vi "PWM2 Init.vi"(5 "DutyCycle":u16, 6 "Precision":u16, 7 "Polarity":u8, 9 "Frequency":u32, 10 "ChannelIndex":u8, 11 "DevHandle":i32) -> (3 "function return":i32)   [LabVIEW 2010, in "usb2pwm.lvlib"]
doc: "int WINAPI PWM2_Init(int DevHandle, unsigned char ChannelIndex,unsigned int Frequency, unsigned char Polarity,unsigned short Precision, unsigned short DutyCycle);"
uses:
  usb2pwm.lvlib
  USB2XXX/trunk/USB2XXX/USB2XXX/vs2019/Release/USB2XXX.dll
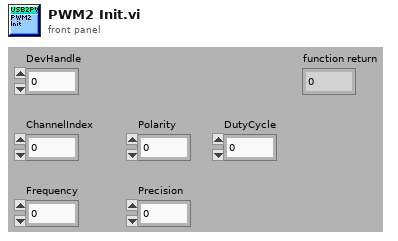
[diagram p1: front panel]
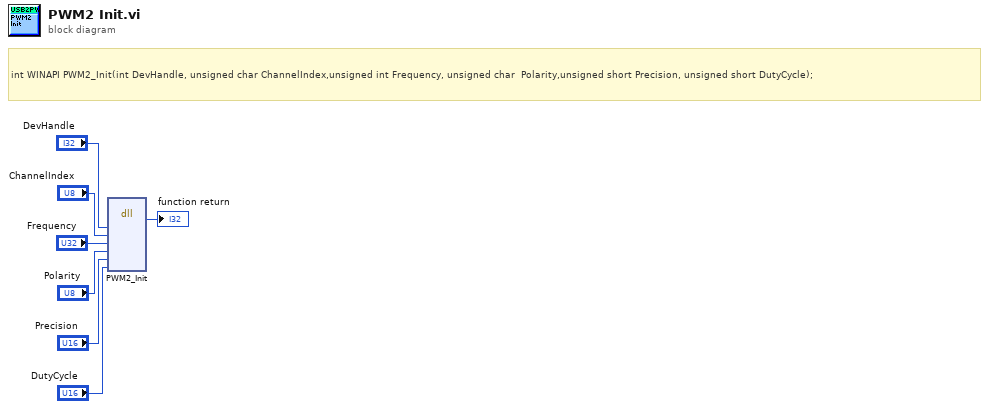
[diagram p0: block diagram]
diagram:
  # "int WINAPI PWM2_Init(int DevHandle, unsigned char ChannelIndex,unsigned int Frequency, unsigned char  Polarity,unsigned short Precision, unsigned short DutyCycle);"
  n1 = dll-call lib="E:/Projects/USB2XXX/trunk/USB2XXX/USB2XXX/vs2019/Release/USB2XXX.*" fn="PWM2_Init"("DevHandle"="DevHandle", "ChannelIndex"="ChannelIndex", "Frequency"="Frequency", "Polarity"="Polarity", "Precision"="Precision", "DutyCycle"="DutyCycle") -> (→"function return":i32)  [unwired: 9 in, 2 out]
